vi "DtCreateCtrTwoEdgeChan.vi"(1 "Start Edge":i32(ring)=752 items=["GateRising"=750, "GateFalling"=751, "ClockRising"=752, "ClockFalling"=753], 2 "Stop Edge":i32(ring)=752 items=["GateRising"=750, "GateFalling"=751, "ClockRising"=752, "ClockFalling"=753], 5 "Board Name":string, 7 "Counter Num":u32, 11 "error in (no error)":errorcluster) -> (4 "Task out":i32, 15 "error out":errorcluster)   [LabVIEW 2022 SP3]
doc: "Creates one or more virtual counter/timer channels that measure the time, in milliseconds, between a specified start edge and stop edge of the counter's clock or gate input signal, and then stops."
uses:
  DtLvLink.lvlib
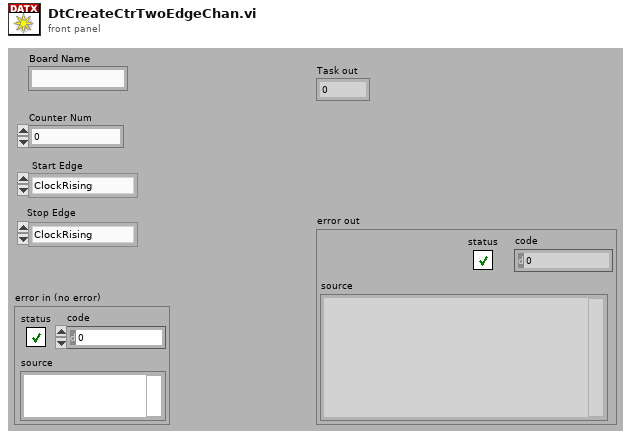
[diagram p1: front panel]
types:
  T1 = enum32{"AnalogInput", "AnalogOutput", "DigitalInput", "DigitalOutput", "Quadrature", "CounterTimer"}
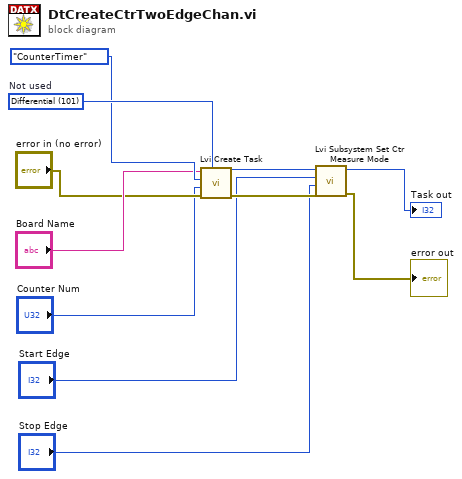
[diagram p0: block diagram]
diagram:
  w11 = 101 items=["SingleEnded"=100, "Differential"=101]  # Not used
  n1 = call "Lvi Create Task.vi"("SEorDiff"=w11, "error in (no error)"="error in (no error)", "SubSysIndex"="Counter Num", "ChanType"=T1."CounterTimer", "BoardName"="Board Name") -> ("error out"=w5:errorcluster, "TaskRef"=w6:i32)  [unwired: 4 in, 1 out]
  n2 = call "Lvi Subsystem Set Ctr Measure Mode.vi"("error in (no error)"=w5, "StopEdge"="Stop Edge", "StartEdge"="Start Edge", "TaskRef"=w6) -> ("error out"=→"error out":errorcluster, "TaskRef out"=→"Task out":i32)  [unwired: 5 in, 1 out]
